vi "数据库更新_B030.vi"(5 "数据":string[](array[string])=["PPPPPP", "1", "1", "1", "1", "1", "1", "1", "1", "100", "100", "100", "200", "200", "200", "300", "300", "300", "300", "300", "300", "300", "300"], 11 "error in (no error)":errorcluster) -> (15 "error out":errorcluster)   [LabVIEW 2013]
panel:
  in  "数据名":string[](array[string])=["weiyi", "本工位完成", "本工位合格", "返工次数", "开始时间", "结束时间", "设备号", "压垫片监控点位移", "压垫片监控点压力", "压垫片压装位移", "压衬套监控点位移", "压衬套监控点压力", "压衬套压装位移", "压轴承监控点位移", "压轴承监控点压力", "压轴承压装位移", "轴承批次号", "衬套批次号", "衬套挡圈批次号", "缓冲垫片批次号"]
  out "连接的字符串":string
  # "CZZ\nWC\nHG\nKSSJ\nJSSJ\nFGCS\nSBID\nDate1\nDate2\nDate3\nDate4\nDate5\nDate6\nDate7\nDate8\nDate9\nDate10"
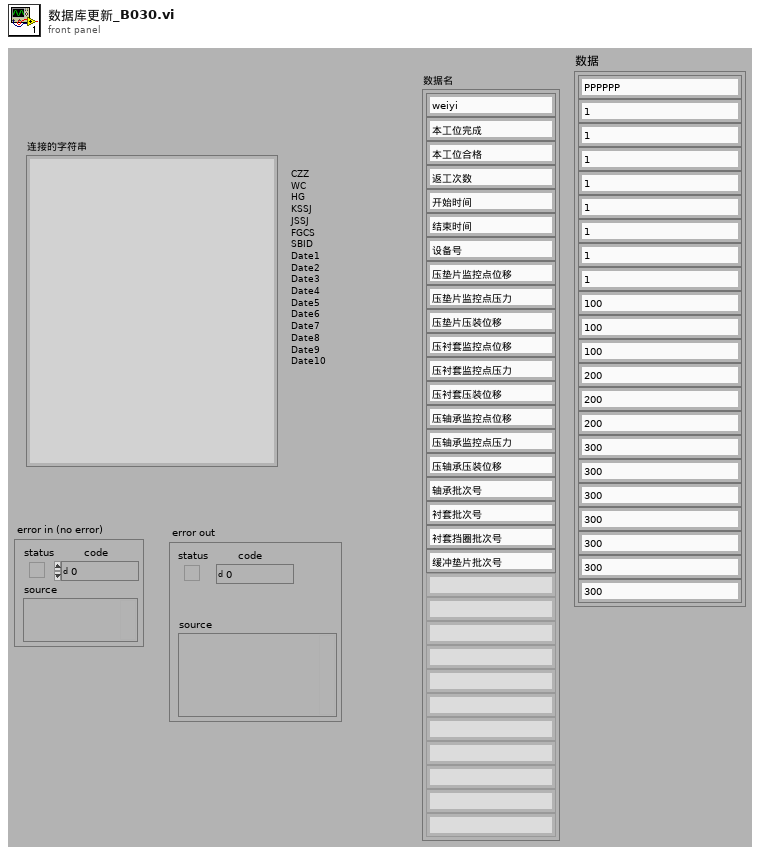
[diagram p1: front panel]
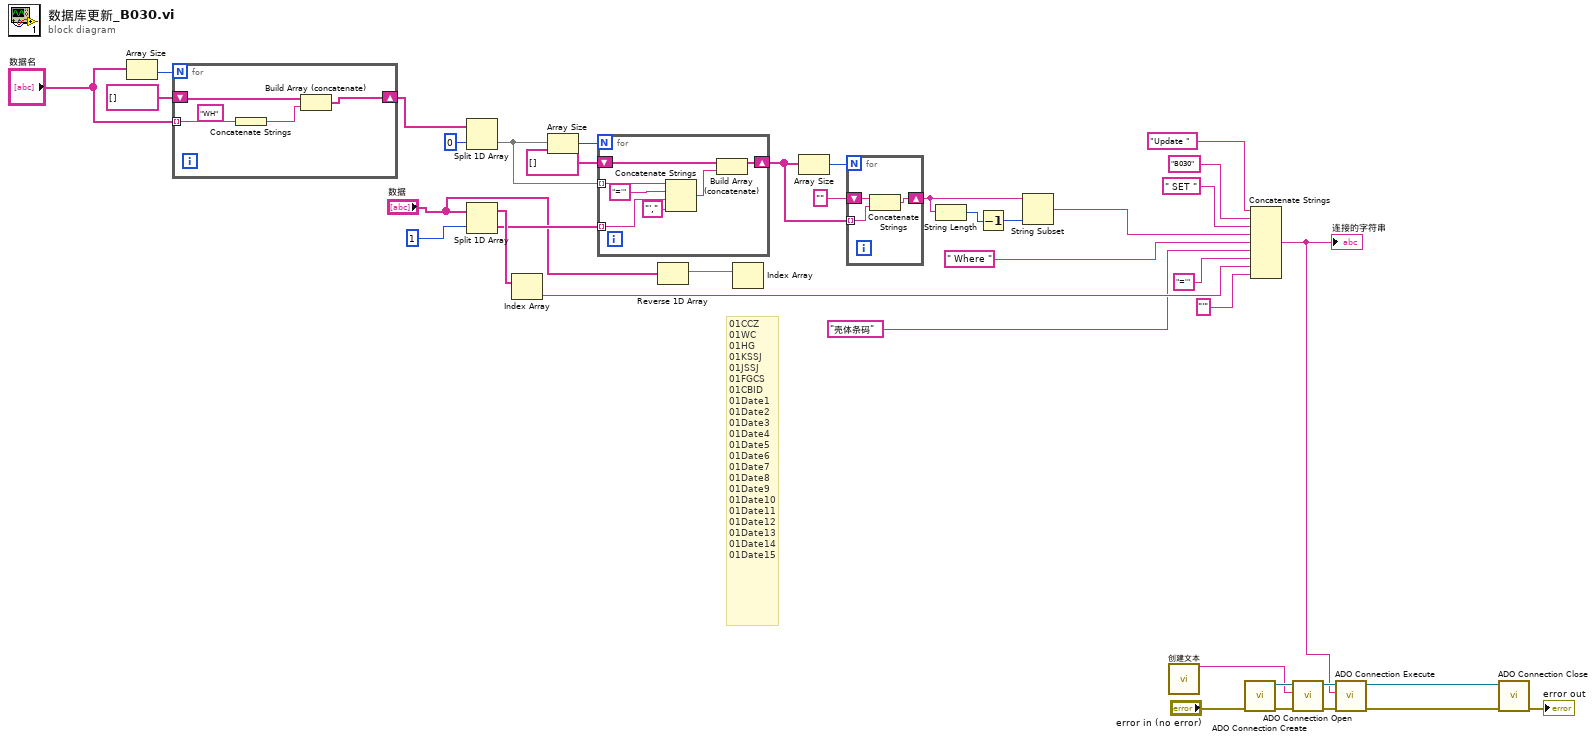
[diagram p0: block diagram]
diagram:
  # "01CCZ\n01WC\n01HG\n01KSSJ\n01JSSJ\n01FGCS\n01CBID\n01Date1\n01Date2\n01Date3\n01Date4\n01Date5\n01Date6\n01Date7\n01Date8\n01Date9\n01Date10\n01Date11\n01Date12\n01Date13\n01Date14\n01Date15"
  n1 = Array Size(array="数据名") -> (size(s)=w10:i32)
  n2 = for {
    N: w10 -> [_]
    tunnel: "数据名" -> [w39] mode=indexing
    shift-right: [w40] -> w8
    shift-left: string[] [] -> [w42]
    (unwired) "WH" ("字符串")
    n3 = Concatenate Strings(w39) -> (w41:string)
    n4 = Build Array (concatenate)(w42, w41) -> (w40:string[])
  }
  n5 = Split 1D Array(array=w8, index=0 ("索引")) -> (second subarray=w26:string[])  [unwired: 1 out]
  n6 = Split 1D Array(array="数据", index=1 ("索引列")) -> (first subarray=w28:string[], second subarray=w25:string[])
  n7 = Index Array(array=w28) -> (element=w13:string)  [unwired: 1 in]
  n8 = Array Size(array=w26) -> (size(s)=w27:i32)
  n9 = for {
    N: w27 -> [_]
    tunnel: w26 -> [w49] mode=indexing
    shift-right: [w46] -> w23
    shift-left: string[] [] -> [w45]
    tunnel: w25 -> [w44] mode=indexing
    n10 = Concatenate Strings(w49, "='" ("字符串"), w44, "'," ("字符串")) -> (w47:string)
    n11 = Build Array (concatenate)(w45, w47) -> (w46:string[])
  }
  n12 = Reverse 1D Array(array="数据") -> (reversed array=w7:string[])
  n13 = Index Array(array=w7) -> ()  [unwired: 1 in, 1 out]
  n14 = Array Size(array=w23) -> (size(s)=w24:i32)
  n15 = for {
    N: w24 -> [_]
    tunnel: w23 -> [w52] mode=indexing
    shift-right: [w51] -> w22
    shift-left: "" -> [w50]
    n16 = Concatenate Strings(w50, w52) -> (w51:string)
  }
  n17 = String Length(string=w22) -> (length=w5:i32)
  n18 = Decrement(x=w5) -> (x-1=w4:i32)
  n19 = String Subset(string=w22, length (rest)=w4) -> (substring=w3:string)  [unwired: 1 in]
  n20 = call "创建文本"() -> ("Result"=w30:string)  [unwired: 14 in, 1 out]
  n21 = call "ADO Connection Create.vi"("error in (no error)"="error in (no error)") -> ("error out"=w37:errorcluster, "ADODB._Connection Out"=w36:refnum<k7>)  [unwired: 9 out]
  n22 = Concatenate Strings("Update " ("字符串"), "B030" ("数据库名"), " SET " ("字符串"), w3, " Where " ("字符串"), "壳体条码" ("索引列名"), "='" ("字符串"), w13, "'" ("字符串")) -> (w6:string)
  "连接的字符串" <- w6
  n23 = call "ADO Connection Open.vi"("error in (no error)"=w37, "ConnectionString"=w30, "ADODB._Connection In"=w36) -> ("error out"=w35:errorcluster, "ADODB._Connection Out"=w34:refnum<k7>)  [unwired: 7 out]
  n24 = call "ADO Connection Execute.vi"("error in (no error)"=w35, "CommandText"=w6, "ADODB._Connection In"=w34) -> ("error out"=w33:errorcluster, "ADODB._Connection Out"=w32:refnum<k7>)  [unwired: 7 out]
  n25 = call "ADO Connection Close.vi"("error in (no error)"=w33, "ADODB._Connection In"=w32) -> ("error out"=→"error out":errorcluster)  [unwired: 9 out]
